vi "Press Button.vi"(0 "GEA2 Reference In":refnum<k24>, 7 "Button":T1=enum."SW201 - My Cycle", 11 "Error In":errorcluster) -> (4 "GEA2 Reference Out":refnum<k24>, 15 "Error Out":errorcluster)   [LabVIEW 2016, in "TL27.lvlib"]
doc: "This VI is used to perform button presses on the HEUI and LEUI."
uses:
  Projects/TL27.lvlib
  type defs/UI Buttons.ctl
  Q:/Common/DLLs/GEA3/GeaCommunication.dll
  Common/DLLs/GEA3/GeaCommunication.dll
  Common/LabVIEW GEA2 Toolkit/LabVIEW_GEA2_Toolkit.lvlibp/type defs/ERD Write Data In.ctl
  Common/LabVIEW GEA2 Toolkit/LabVIEW_GEA2_Toolkit.lvlibp/type defs/Data Type.ctl
  Common/LabVIEW GEA2 Toolkit/LabVIEW_GEA2_Toolkit.lvlibp/type defs/Source_Destination.ctl
  Common/LabVIEW GEA2 Toolkit/LabVIEW_GEA2_Toolkit.lvlibp
panel:
  in  "Standalone?":bool
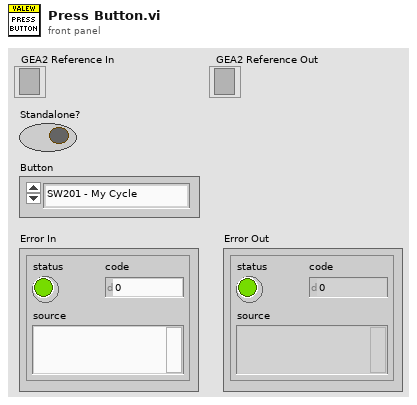
[diagram p1: front panel]
types:
  T1 = typedef "TL27.lvlib/UI Buttons.ctl" = enum16{"Switch Off", "SW201 - My Cycle", "SW202 - Delay Wash", "SW203 - Extra Rinse", "SW204 - Signal / Volume", "SW205 - Spin", "SW206 - Deep Rinse / Fab Soft", "SW207 - Soil", "SW208 - Auto Soak", "SW209 - Temp", "SW210 - Warm Rinse", "SW211 - Deep Fill", "SW212 - Stain Remover", "SW213 - Power", "SW222 - Control Lock", "SW214 - Start / Pause", "SW301 - Start/Pause LE", "SW302 - Option Button LE", "SW201/212 - Bulk Flush"}
  T2 = typedef "LabVIEW_GEA2_Toolkit.lvlibp/Source_Destination.ctl" = cluster{"Source":u8, "Destination":u8}
  T3 = typedef "LabVIEW_GEA2_Toolkit.lvlibp/ERD Write Data In.ctl" = cluster{"ERD Number":u16, "Data Type":T4, "Data":string}
  T4 = typedef "LabVIEW_GEA2_Toolkit.lvlibp/Data Type.ctl" = enum16{"string", "boolean", "uint8_t", "uint16_t", "uint32_t", "uint64_t", "int8_t", "int16_t", "int32_t", "int64_t"}
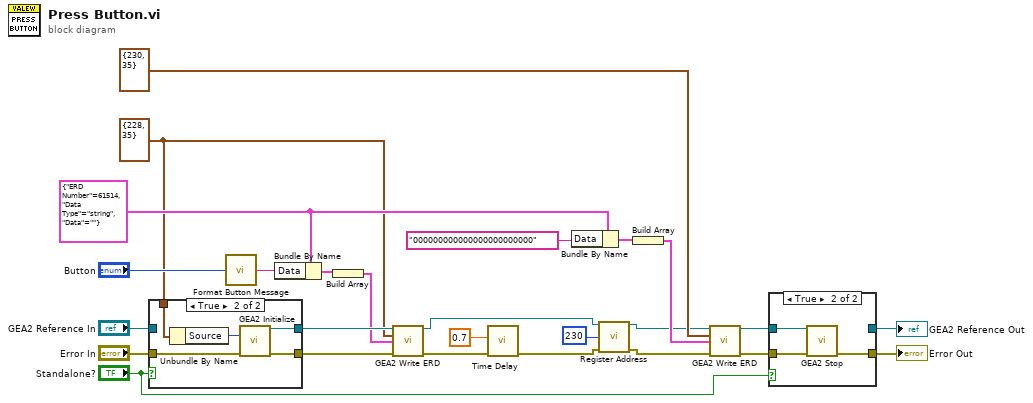
[diagram p0: block diagram]
diagram:
  w7 = T2 {"Source"=228, "Destination"=35} ("GEA Inputs")
  w8 = T3 {"ERD Number"=61514, "Data Type"=enum."string", "Data"=""} ("ERD Write Data In")
  n1 = case shown="True" "Standalone?" {
    tunnel: "Error In" -> [w27 w33]
    tunnel: [w27 w32] -> w19
    tunnel: "GEA2 Reference In" -> [w28 _]
    tunnel: [w28 w31] -> w17
    tunnel: w7 -> [_ w29]
    frame False {
    }
    frame True {
      n2 = Unbundle By Name(w29) -> ("Source"=w30:u8)
      n3 = call "GEA2 Initialize.vi"("Source Address"=w30, "error in"=w33) -> ("GEA2 Reference Out"=w31:refnum<k24>, "error out"=w32:errorcluster)  [unwired: 11 in, 1 out]
    }
  }
  n4 = call "Format Button Message.vi"("Switch"="Button") -> ("Switch Message"=w16:string)  [unwired: 14 in]
  n5 = Bundle By Name(cluster=w8, "Data"=w16) -> (w15:T3)
  n6 = Build Array(w15) -> (w14:T3[])
  n7 = call "GEA2 Write ERD.vi"("GEA2 Reference In"=w17, "GEA Inputs"=w7, "Write ERD List"=w14, "Error In"=w19) -> ("GEA2 Reference Out"=w2:refnum<k24>, "Error Out"=w18:errorcluster)  [unwired: 9 in, 1 out]
  n8 = call "Time Delay"("error in (no error)"=w18, "Delay Time (s)"=0.7) -> ("error out"=w4:errorcluster)  [unwired: 9 in]
  n9 = Bundle By Name(cluster=w8, "Data"="000000000000000000000000" ("Message")) -> (w10:T3)
  n10 = call "Register Address.vi"("GEA2 Reference In"=w2, "Address"=u8 230 ("Source"), "Error In"=w4) -> ("GEA2 Reference Out"=w1:refnum<k24>, "Error Out"=w3:errorcluster)  [unwired: 11 in]
  n11 = Build Array(w10) -> (w9:T3[])
  n12 = call "GEA2 Write ERD.vi"("GEA2 Reference In"=w1, "GEA Inputs"=T2 {"Source"=230, "Destination"=35}, "Write ERD List"=w9, "Error In"=w3) -> ("GEA2 Reference Out"=w13:refnum<k24>, "Error Out"=w12:errorcluster)  [unwired: 9 in, 1 out]
  n13 = case shown="True" "Standalone?" {
    tunnel: [w34 w38] -> w22
    tunnel: w13 -> [w35 w37]
    tunnel: [w35 _] -> w21
    tunnel: w12 -> [w34 w36]
    frame False {
    }
    frame True {
      n14 = call "GEA2 Stop.vi"("GEA2 Reference In"=w37, "Error In"=w36) -> ("Error Out"=w38:errorcluster)  [unwired: 13 in]
    }
  }
  "Error Out" <- w22
  "GEA2 Reference Out" <- w21
